vi "stable settings.vi"() -> ()   [LabVIEW 2016]
doc: "when a number stable current run type is selected this pop up will let user inportant values for correct measurements"
panel:
  in  "Charge State":dbl=3.0
  in  "stop":bool
  in  "1st offset current(nA/V)":dbl=500.0
  in  "2nd offset current (nA/V)":dbl=1000.0
  in  "field change wait(s)":u32=5
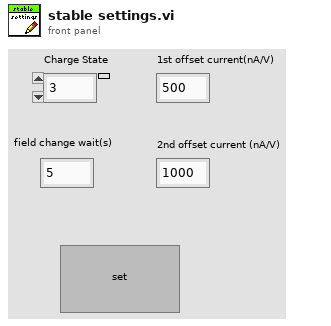
[diagram p1: front panel]
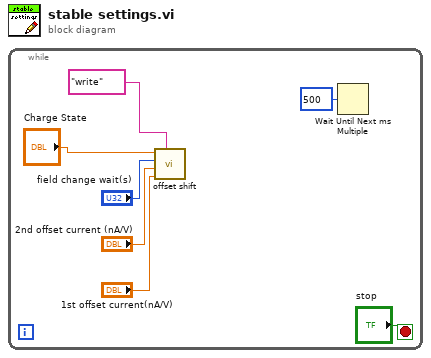
[diagram p0: block diagram]
diagram:
  n1 = while {
    stop <- "stop" stop-if-true
    n2 = call "offset shift.vi"("read writ"="write", "na/V"="1st offset current(nA/V)", "na/V 2"="2nd offset current (nA/V)", "field change wait(s)"="field change wait(s)", "charge state"="Charge State") -> ()  [unwired: 3 in, 4 out]
    n3 = Wait Until Next ms Multiple(millisecond multiple=u32 500) -> ()  [unwired: 1 out]
  }
